vi "Initialize.vi"(8 "error in (no error)":errorcluster, 11 "GW-Stop-Cmd in":refnum<class "GW-Stop-Cmd.lvclass">) -> (0 "error out":errorcluster, 3 "GW-Stop-Cmd out":refnum<class "GW-Stop-Cmd.lvclass">)   [LabVIEW 2013, in "GW-Stop-Cmd.lvclass"]
uses:
  GW-Stop-Cmd.lvclass
  States/GW-Stopping-State/GW-Stopping-State.lvclass
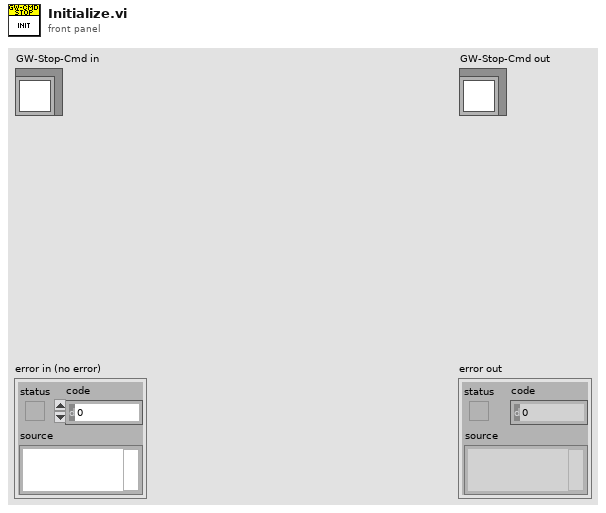
[diagram p1: front panel]
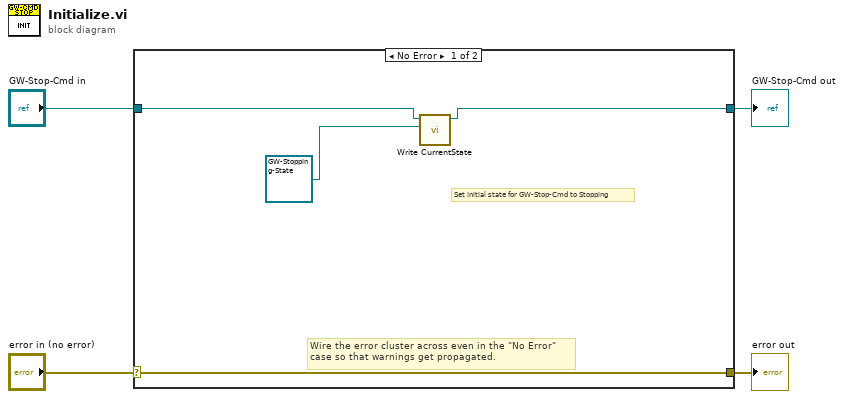
[diagram p0: block diagram]
diagram:
  n1 = case shown="No Error" "error in (no error)" {
    selector: "error in (no error)" -> [w8 w10]
    tunnel: [w8 w10] -> w3
    tunnel: [w6 w9] -> w1
    tunnel: "GW-Stop-Cmd in" -> [w7 w9]
    frame No Error {
      # "Set initial state for GW-Stop-Cmd to Stopping"
      # "Wire the error cluster across even in the \"No Error\"\ncase so that warnings get propagated."
      n2 = call-dynamic "Write CurrentState.vi"("State.lvclass"=refnum<class "GW-Stopping-State.lvclass"> refnum ("GW-Stopping-State.lvclass"), "Command in"=w7) -> ("Command out"=w6:refnum<class "GW-Stop-Cmd.lvclass">)  [unwired: 8 in, 1 out]
    }
    frame Error {
    }
  }
  "error out" <- w3
  "GW-Stop-Cmd out" <- w1
